vi "Exit.vi"(8 "error in (no error)":errorcluster, 11 "Old State":refnum<class "Init_cls.lvclass">) -> (0 "error out":errorcluster, 3 "New State":refnum<class "Init_cls.lvclass">)   [LabVIEW 2025, in "Demo_States.lvlib" / "Init_cls.lvclass"]
doc: "This is an abstract method. Override this method to define the behavior when you leave the state."
uses:
  Init_cls.lvclass
  Demo_States/Demo_States.lvclass
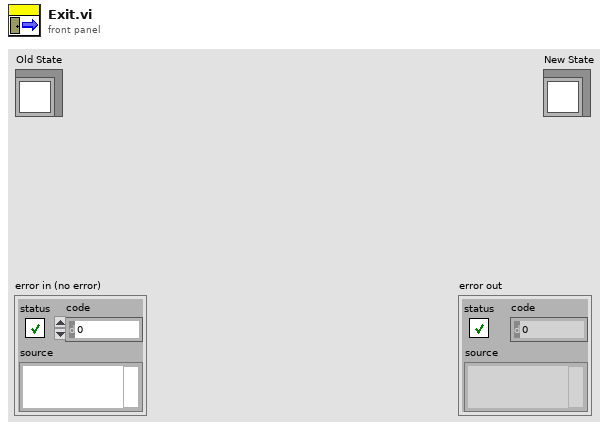
[diagram p1: front panel]
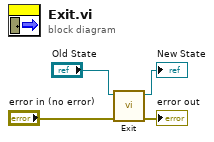
[diagram p0: block diagram]
diagram:
  n1 = call-parent "Exit.vi"("error in (no error)"="error in (no error)", "Old State"="Old State") -> ("error out"=→"error out":errorcluster, "New State"=→"New State":refnum<class "Init_cls.lvclass">)  [unwired: 8 in]
